vi "WaitOn WaitForNotifier.vi"(8 "error in (no error)":errorcluster, 9 "timeout in ms (-1)":i32=-1, 10 "Wait until finished?":bool, 11 "notifier":refnum<notifier>) -> (0 "error out":errorcluster, 3 "timed out?":bool)   [LabVIEW 2021, in "BluePlot.lvlib"]
uses:
  BluePlot.lvlib
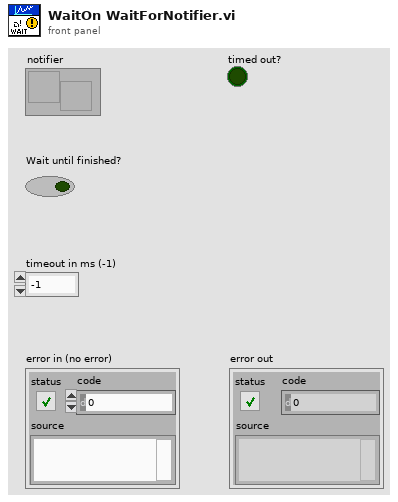
[diagram p1: front panel]
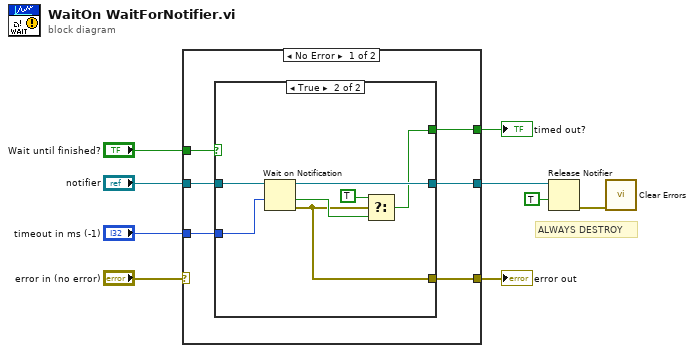
[diagram p0: block diagram]
diagram:
  # "ALWAYS DESTROY"
  n1 = case shown="No Error" "error in (no error)" {
    selector: "error in (no error)" -> [_ w25]
    tunnel: "Wait until finished?" -> [w15 _]
    tunnel: "timeout in ms (-1)" -> [w14 _]
    tunnel: "notifier" -> [w13 w24]
    tunnel: [w12 _] -> w6
    tunnel: [w10 w25] -> w4
    tunnel: [w11 w24] -> w2
    frame No Error {
      n2 = case shown="True" w15 {
        tunnel: w14 -> [_ w23]
        tunnel: w13 -> [w16 w22]
        tunnel: [w16 w21] -> w11
        tunnel: [_ w18] -> w12
        tunnel: [_ w17] -> w10
        frame False {
        }
        frame True {
          n3 = Wait on Notification(notifier=w22, timeout in ms (-1)=w23) -> (notifier out=w21:refnum<notifier>, timed out?=w19:bool, error out=w17:errorcluster)  [unwired: 2 in, 1 out]
          n4 = Select(t=TRUE ("timed out?"), s=w17, f=w19) -> (s? t:f=w18:bool)
        }
      }
    }
    frame Error {
    }
  }
  "error out" <- w4
  "timed out?" <- w6
  n5 = Release Notifier(notifier=w2, force destroy? (F)=TRUE) -> (error out=w3:errorcluster)  [unwired: 1 in, 2 out]
  n6 = call <vilib>:"Clear Errors.vi"("error in (no error)"=w3) -> ()  [unwired: 5 in, 2 out]
